vi "RenameAllFoldersToLower.vi"() -> ()   [LabVIEW 2024]
panel:
  out "current folder":string
  out "error out":errorcluster
  out "Array":path[](array[path])
  in  "Folder Path":path=path "D:/Comics/Marvel"
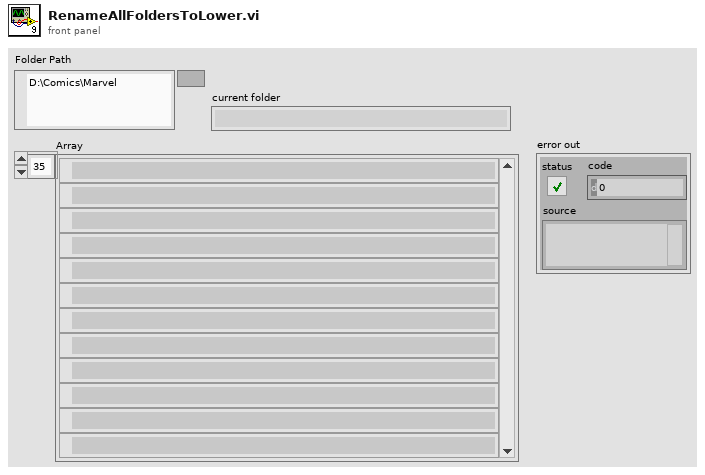
[diagram p1: front panel]
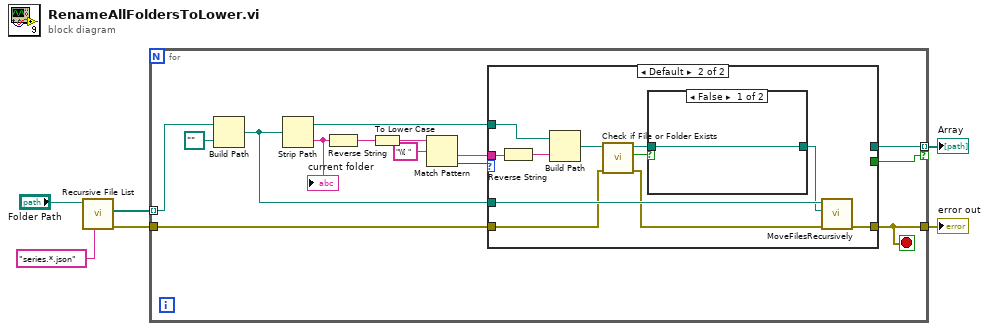
[diagram p0: block diagram]
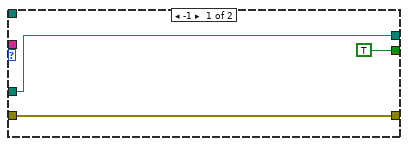
[diagram p2: hidden frame]
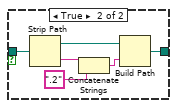
[diagram p3: hidden frame]
diagram:
  n1 = call <vilib>:"Recursive File List.vi"("pattern"="series.*.json", "Folder Path"="Folder Path") -> ("error out"=w3:errorcluster, "All Files in Dir"=w4:path[])  [unwired: 5 in, 3 out]
  n2 = for {
    tunnel: w4 -> [w12] mode=indexing
    tunnel: w3 -> [w13]
    tunnel: [w10] -> w2 mode=indexing if=w8
    tunnel: [w7] -> w1
    stop <- w7 stop-if-true
    n3 = Build Path(base path=w12, name or relative path=path "..") -> (appended path=w11:path)
    n4 = Strip Path(path=w11) -> (stripped path=w14:path, name=w19:string)
    "current folder" <- w19
    n5 = Reverse String(1:w19) -> (0:w18:string)
    n6 = To Lower Case(string=w18) -> (all lower case string=w17:string)
    n7 = Match Pattern(string=w17, regular expression="\\[ ") -> (after substring=w15:string, offset past match=w9:i32)  [unwired: 1 in, 2 out]
    n8 = case shown="Default" w9 {
      tunnel: w15 -> [_ w34]
      tunnel: w14 -> [_ w32]
      tunnel: w13 -> [w23 w28]
      tunnel: w11 -> [w22 w31]
      tunnel: [w22 _] -> w10
      tunnel: [w23 w30] -> w7
      tunnel: [TRUE _] -> w8
      frame -1 {
      }
      frame Default {
        n9 = Reverse String(1:w34) -> (0:w33:string)
        n10 = Build Path(base path=w32, name or relative path=w33) -> (appended path=w29:path)
        n11 = call <vilib>:"Check if File or Folder Exists.vi"("error in (no error)"=w28, "path"=w29) -> ("error out"=w27:errorcluster, "file or folder exists?"=w26:bool, "dup path"=w25:path)  [unwired: 7 in]
        n12 = case shown="False" w26 {
          tunnel: w25 -> [w35 w41]
          tunnel: [w35 w38] -> w24
          frame False {
          }
          frame True {
            n13 = Strip Path(path=w41) -> (stripped path=w37:path, name=w40:string)
            n14 = Concatenate Strings(w40, ".2" ("string")) -> (w36:string)
            n15 = Build Path(base path=w37, name or relative path=w36) -> (appended path=w38:path)
          }
        }
        n16 = call "MoveFilesRecursively.vi"("error in"=w27, "Dest Path"=w24, "Source Path"=w31) -> ("error out"=w30:errorcluster)  [unwired: 8 in]
      }
    }
  }
  "Array" <- w2
  "error out" <- w1
